vi "Fetch Measurement (Trace Data).vi"(8 "error in (no error)":errorcluster, 10 "Select Trace (1: Trace 1)":u16(ring)=1 items=["Trace 1"=1, "Trace 2"=2, "Trace 3"=3], 11 "VISA resource name":refnum<visa-resource-name>) -> (0 "error out":errorcluster, 1 "Log Plot":cluster{dbl[], dbl[]}(graph), 2 "Measured Values":dbl[](array[numeric]) format="%#.6g", 3 "VISA resource name out":refnum<visa-resource-name>)   [LabVIEW 2014, in "Agilent ESA PSA Series.lvlib"]
doc: "Returns the results of the last measurement (Trace Data) and does not initiate data acquisition.\n\n<B>Note:</B> \n\nThis VI is only valid for the Log Plot functionality of the Phase noise personality."
uses:
  Agilent ESA PSA Series.lvlib
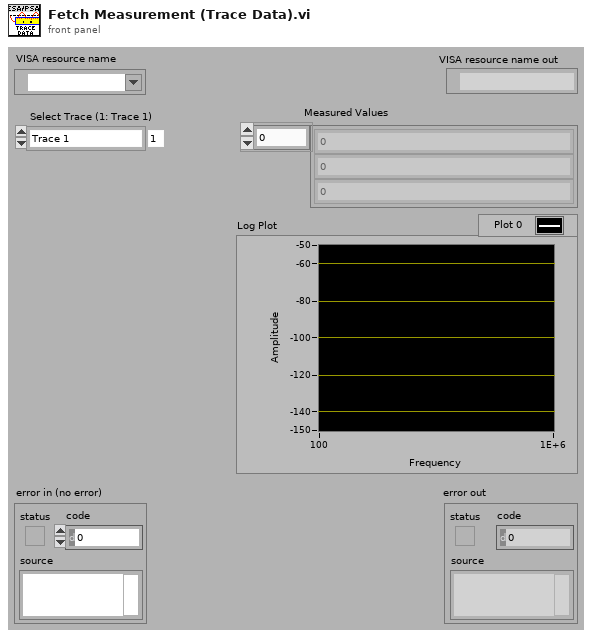
[diagram p1: front panel]
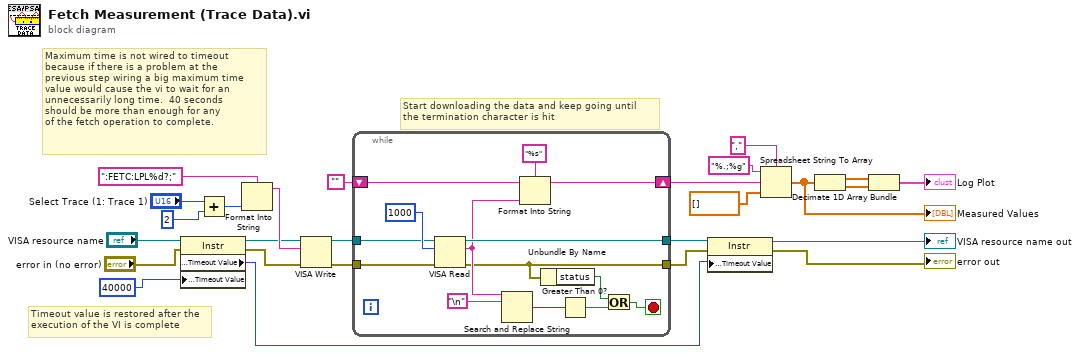
[diagram p0: block diagram]
diagram:
  # "Maximum time is not wired to timeout\nbecause if there is a problem at the\nprevious step wiring a big maximum time\nvalue would cause the vi to wait for an\nunnecessarily long time.  40 seconds\nshould be more than enough for any\nof the fetch operation to complete."
  # "Timeout value is restored after the\nexecution of the VI is complete"
  # "Start downloading the data and keep going until\nthe termination character is hit"
  n1 = property on="Property Node" class="Instr"(reference="VISA resource name", error in="error in (no error)", "General Settings:Timeout Value"=u32 40000) -> (reference out=w21:refnum<visa-resource-name>, error out=w22:errorcluster, "General Settings:Timeout Value"=w18:u32)
  n2 = Add(x="Select Trace (1: Trace 1)", y=u16 2) -> (x+y=w8:u16)
  n3 = Format Into String(format string=":FETC:LPL%d?;" ("string (\"\")"), w8) -> (resulting string=w25:string)  [unwired: 2 in, 1 out]
  n4 = VISA Write(VISA resource name=w21, write buffer=w25, error in (no error)=w22) -> (VISA resource name out=w12:refnum<visa-resource-name>, error out=w11:errorcluster)  [unwired: 1 out]
  n5 = while {
    tunnel: [w39] -> w20
    tunnel: [w27] -> w19
    tunnel: w12 -> [w38]
    tunnel: w11 -> [w37]
    shift-right: [w33] -> w9
    shift-left: "" -> [w32]
    stop <- w28 stop-if-true
    n6 = VISA Read(VISA resource name=w38, byte count=u32 1000, error in (no error)=w37) -> (VISA resource name out=w39:refnum<visa-resource-name>, read buffer=w34:string, error out=w27:errorcluster)  [unwired: 1 out]
    n7 = Search and Replace String(input string=w34, search string="\n") -> (number of replacements=w35:i32)  [unwired: 6 in, 3 out]
    n8 = Format Into String(format string="%s", initial string=w32, w34) -> (resulting string=w33:string)  [unwired: 1 in, 1 out]
    n9 = Unbundle By Name(w27) -> ("status"=w30:bool)
    n10 = Greater Than 0?(x=w35) -> (x > 0?=w29:bool)
    n11 = Or(x=w30, y=w29) -> (x .or. y?=w28:bool)
  }
  n12 = property on="Property Node" class="Instr"(reference=w20, error in=w19, "General Settings:Timeout Value"=w18) -> (reference out=→"VISA resource name out":refnum<visa-resource-name>, error out=→"error out":errorcluster)
  n13 = Spreadsheet String To Array(delimiter (Tab)=",", format string="%.;%g", spreadsheet string=w9, array type (2D Dbl)=dbl[] []) -> (array=w4:dbl[])
  "Measured Values" <- w4
  n14 = Decimate 1D Array(w4) -> (w3:dbl[], w2:dbl[])
  n15 = Bundle(w3, w2) -> (→"Log Plot":cluster{dbl[], dbl[]})  [unwired: 1 in]
